vi "Select Panther Scan File to load.vi"(11 "PantherScan bin Files":path[](array[path])) -> (2 "Continue?":bool, 3 "Panther Scan Selected":path)   [LabVIEW 2019, in "Panther Dashboard.lvlib" / "Project.lvclass"]
uses:
  Project.lvclass
panel:
  in  "Panther Scans":i32(listbox)
  out "Info":string
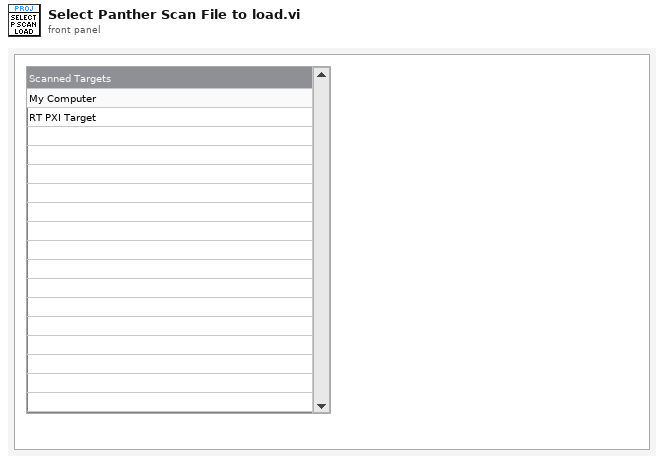
[diagram p1: front panel]
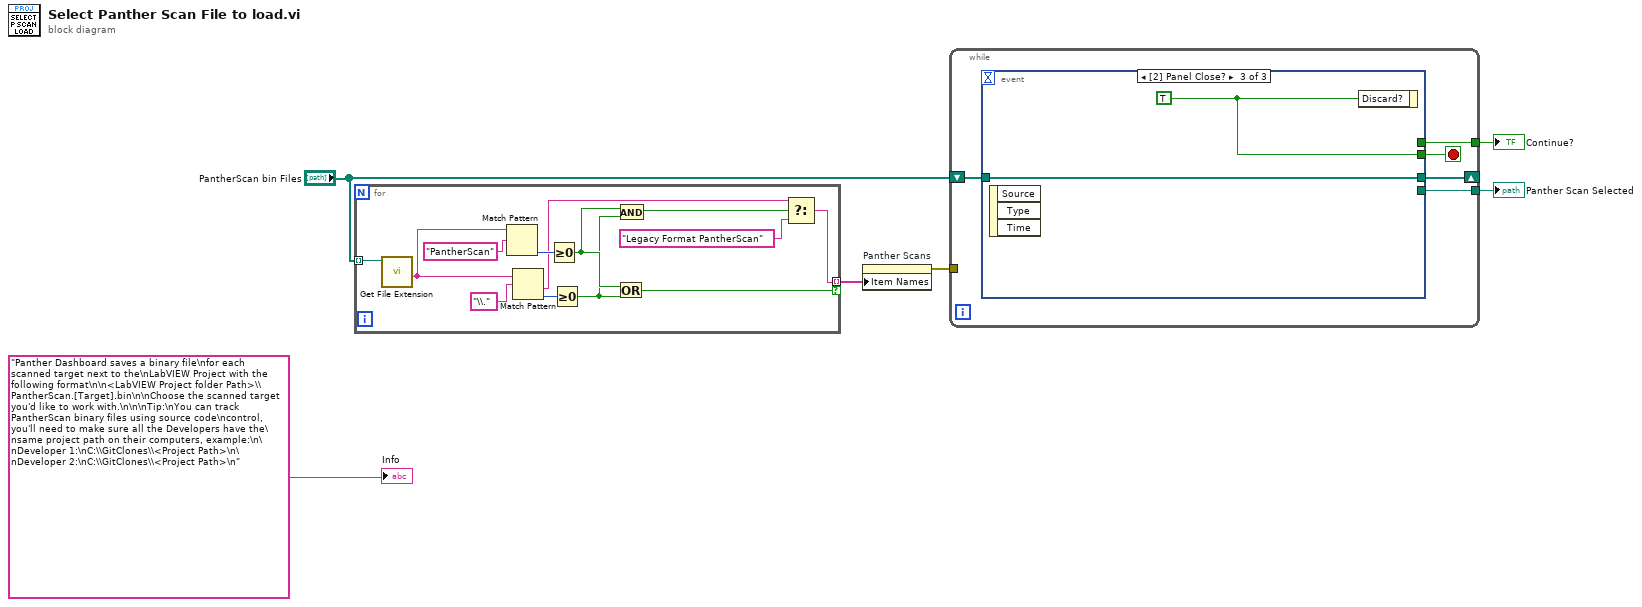
[diagram p0: block diagram]
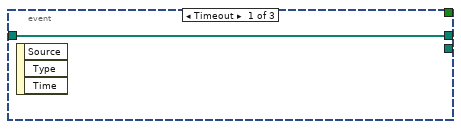
[diagram p2: hidden frame]
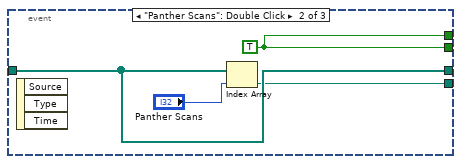
[diagram p3: hidden frame]
diagram:
  n1 = for {
    tunnel: [w14] -> w2 mode=indexing if=w9
    tunnel: "PantherScan bin Files" -> [w19] mode=indexing
    n2 = call <vilib>:"Get File Extension.vi"("file"=w19) -> ("filename without extension"=w8:string)  [unwired: 6 in, 4 out]
    n3 = Match Pattern(string=w8, regular expression="PantherScan") -> (offset past match=w15:i32)  [unwired: 1 in, 3 out]
    n4 = Match Pattern(string=w8, regular expression="\\.") -> (after substring=w12:string, offset past match=w17:i32)  [unwired: 1 in, 2 out]
    n5 = Greater Or Equal To 0?(x=w15) -> (x >= 0?=w11:bool)
    n6 = Greater Or Equal To 0?(x=w17) -> (x >= 0?=w10:bool)
    n7 = Or(x=w11, y=w10) -> (x .or. y?=w9:bool)
    n8 = And(x=w11, y=w10) -> (x .and. y?=w13:bool)
    n9 = Select(t=w12, s=w13, f="Legacy Format PantherScan") -> (s? t:f=w14:string)
  }
  n10 = property on="Panther Scans" class="LstBox (strict)"("Item Names"=w2) -> (error out=w6:errorcluster)  [unwired: 2 in, 1 out]
  n11 = while {
    tunnel: [w22] -> w5
    tunnel: w6 -> [_]
    tunnel: [w21] -> w3
    shift-right: [w20] -> _
    shift-left: "PantherScan bin Files" -> [w23]
    stop <- w24 stop-if-true
    n12 = event shown="[2] Panel Close?" {
      selector: _ -> [_ _ _]
      dyn-events: _ -> [_ _ _]
      timeout: _ -> [_ _ _]
      tunnel: [_ w26 w31] -> w24
      tunnel: w23 -> [w25 w28 w30]
      tunnel: [_ w27 _] -> w22
      tunnel: [_ w26 _] -> w21
      tunnel: [w25 w28 w30] -> w20
      event Timeout {
        n13 = event-data() -> ()  [unwired: 1 in, 3 out]
      }
      event "Panther Scans": Double Click {
        w26 = TRUE ("Discard?")
        n14 = event-data() -> ()  [unwired: 1 in, 3 out]
        n15 = Index Array(array=w28, index="Panther Scans") -> (element=w27:path)
      }
      event Panel Close? {
        w31 = TRUE ("Discard?")
        n16 = event-data() -> ()  [unwired: 1 in, 3 out]
        n17 = event-data("Discard?"=w31) -> ()  [unwired: 1 in, 1 out]
      }
    }
  }
  "Continue?" <- w3
  "Panther Scan Selected" <- w5
  "Info" <- "Panther Dashboard saves a binary file\nfor each scanned target next to the\nLabVIEW Project with the following format\n\n<LabVIEW Project folder Path>\\PantherScan.[Target].bin\n\nChoose the scanned target you'd like to work with.\n\n\nTip:\nYou can track PantherScan binary files using source code\ncontrol, you'll need to make sure all the Developers have the\nsame project path on their computers, example:\n\nDeveloper 1:\nC:\\GitClones\\<Project Path>\n\nDeveloper 2:\nC:\\GitClones\\<Project Path>\n" ("String")
